vi "parse_results_for_max.vi"(11 "all file in":path=path "O:/DSG/Tyler/EIC/DIRC/results/BA1_only_t2_2026-04-01.csv") -> (3 "max file out":path)   [LabVIEW 2024]
uses:
  d8221273-8729-4a0a-b800-230671b48b45.vi
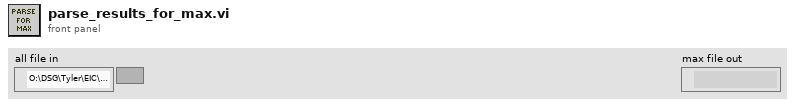
[diagram p1: front panel]
types:
  T1 = enum16{"open", "replace", "create", "open or create", "replace or create", "replace or create with confirmation"}
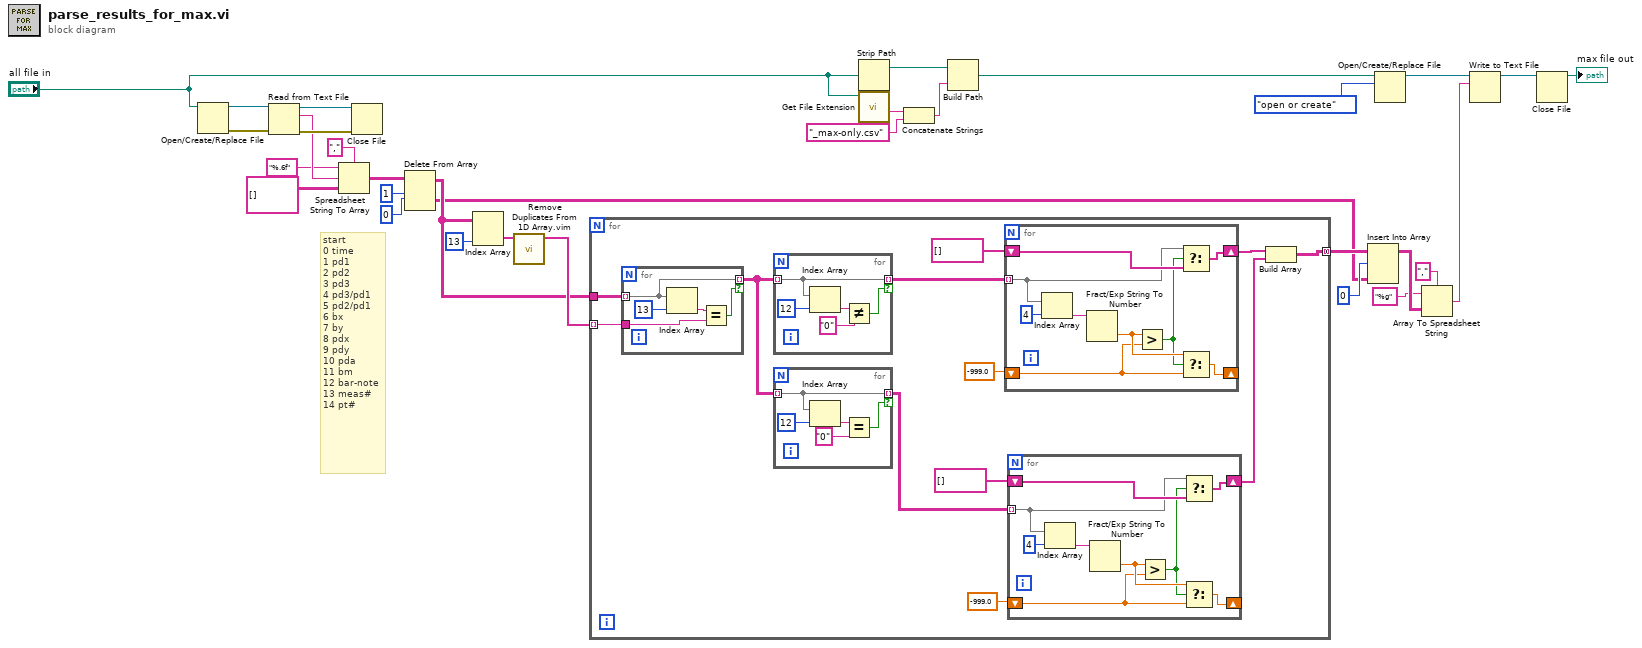
[diagram p0: block diagram]
diagram:
  # "start\n0 time\n1 pd1\n2 pd2\n3 pd3\n4 pd3/pd1\n5 pd2/pd1\n6 bx\n7 by\n8 pdx\n9 pdy\n10 pda\n11 bm\n12 bar-note\n13 meas#\n14 pt#"
  n1 = Open/Create/Replace File(file path (use dialog)="all file in") -> (refnum out=w32:refnum<file>, error out=w30:errorcluster)  [unwired: 5 in, 1 out]
  n2 = Read from Text File(file (use dialog)=w32, error in=w30) -> (refnum out=w31:refnum<file>, text=w28:string, error out=w29:errorcluster)  [unwired: 2 in, 1 out]
  n3 = Spreadsheet String To Array(delimiter (Tab)=",", format string="%.6f", spreadsheet string=w28, array type (2D Dbl)=string[][] []) -> (array=w19:string[][])
  n4 = Close File(refnum=w31, error in=w29) -> ()  [unwired: 2 out]
  n5 = Delete From Array(array=w19, length=1, index (row)=0) -> (deleted portion=w15:string[][], array with subset deleted=w18:string[][])  [unwired: 1 in]
  n6 = Index Array(array=w18, index (col)=13 ("disabled index (col)")) -> (element=w23:string[])  [unwired: 1 in]
  n7 = call "Remove Duplicates From 1D Array.vim"("array"=w23) -> ("array with duplicates removed"=w22:string[])  [unwired: 10 in]
  n8 = for {
    tunnel: w22 -> [w43] mode=indexing
    tunnel: w18 -> [w44]
    tunnel: [w34] -> w17 mode=concatenating
    n9 = for {
      tunnel: w44 -> [w74] mode=indexing
      tunnel: [w74] -> w42 mode=indexing if=w73
      tunnel: w43 -> [w75]
      n10 = Index Array(array=w74, index=13) -> (element=w76:string)
      n11 = Equal?(x=w76, y=w75) -> (x = y?=w73:bool)
    }
    n12 = for {
      tunnel: w42 -> [w71] mode=indexing
      tunnel: [w71] -> w41 mode=indexing if=w70
      n13 = Index Array(array=w71, index=12) -> (element=w69:string)
      n14 = Not Equal?(x=w69, y="0") -> (x != y?=w70:bool)
    }
    n15 = for {
      tunnel: w42 -> [w66] mode=indexing
      tunnel: [w66] -> w40 mode=indexing if=w65
      n16 = Index Array(array=w66, index=12) -> (element=w64:string)
      n17 = Equal?(x=w64, y="0") -> (x = y?=w65:bool)
    }
    n18 = for {
      tunnel: w41 -> [w45] mode=indexing
      shift-right: [w49] -> _
      shift-left: -999.0 -> [w50]
      shift-right: [w48] -> w35
      shift-left: string[] [] -> [w47]
      n19 = Index Array(array=w45, index=4) -> (element=w52:string)
      n20 = Fract/Exp String To Number(string=w52) -> (number=w51:dbl)  [unwired: 3 in, 1 out]
      n21 = Greater?(x=w51, y=w50) -> (0:w46:bool)
      n22 = Select(t=w45, s=w46, f=w47) -> (s? t:f=w48:string[])
      n23 = Select(t=w51, s=w46, f=w50) -> (s? t:f=w49:dbl)
    }
    n24 = for {
      tunnel: w40 -> [w54] mode=indexing
      shift-right: [w58] -> _
      shift-left: -999.0 -> [w59]
      shift-right: [w57] -> w33
      shift-left: string[] [] -> [w56]
      n25 = Index Array(array=w54, index=4) -> (element=w61:string)
      n26 = Fract/Exp String To Number(string=w61) -> (number=w60:dbl)  [unwired: 3 in, 1 out]
      n27 = Greater?(x=w60, y=w59) -> (0:w55:bool)
      n28 = Select(t=w54, s=w55, f=w56) -> (s? t:f=w57:string[])
      n29 = Select(t=w60, s=w55, f=w59) -> (s? t:f=w58:dbl)
    }
    n30 = Build Array(w35, w33) -> (w34:string[][])
  }
  n31 = Strip Path(path="all file in") -> (stripped path=w11:path)  [unwired: 1 out]
  n32 = call <vilib>:"Get File Extension.vi"("file"="all file in") -> ("filename without extension"=w13:string)  [unwired: 6 in, 4 out]
  n33 = Concatenate Strings(w13, "_max-only.csv" ("string")) -> (w10:string)
  n34 = Build Path(base path=w11, name or relative path=w10) -> (appended path=w6:path)
  n35 = Insert Into Array(array=w17, index (row)=0, new element=w15) -> (w9:string[][])  [unwired: 1 in]
  n36 = Open/Create/Replace File(file path (use dialog)=w6, operation (0:open)=T1."open or create") -> (refnum out=w5:refnum<file>)  [unwired: 4 in, 2 out]
  n37 = Array To Spreadsheet String(delimiter (Tab)=",", array=w9, 3:"%g" ("format string")) -> (spreadsheet string=w3:string)
  n38 = Write to Text File(file (use dialog)=w5, text=w3) -> (refnum out=w4:refnum<file>)  [unwired: 2 in, 2 out]
  n39 = Close File(refnum=w4) -> (path=→"max file out":path)  [unwired: 1 in, 1 out]
